vi "Write Status.vi"(5 "Username":string, 6 "Password":string, 7 "Address":string, 8 "Error In":errorcluster) -> (0 "Error Out":errorcluster)   [LabVIEW 2018, in "Tests.lvlib" / "SFTP File.lvlib"]
uses:
  SFTP File.lvlib
  src/Toolkit/SFTP File/Type Definitions/Open Options.ctl
  src/Toolkit/SFTP Attributes/Support/Create from SFTP File.vi
  src/Toolkit/SFTP Attributes/Support/Destroy to SFTP File.vi
  <vilib>/addons/_JKI Toolkits/Caraya/classes/Test/Test.lvclass
  <vilib>/addons/_JKI Toolkits/Caraya/classes/Assert/Assert.lvclass
  src/Toolkit/SFTP File/SFTP File.lvclass
  src/Toolkit/SFTP Attributes/SFTP Attributes.lvclass
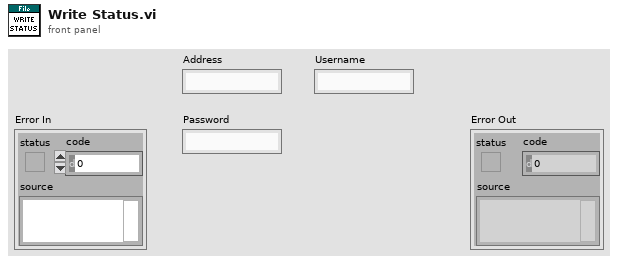
[diagram p1: front panel]
types:
  T1 = typedef "Toolkit.lvlib/SFTP File.lvclass/Open Options.ctl" = cluster{"Read":bool, "Write":bool, "Append":bool, "Create":bool, "Truncate":bool, "Exclude":bool}
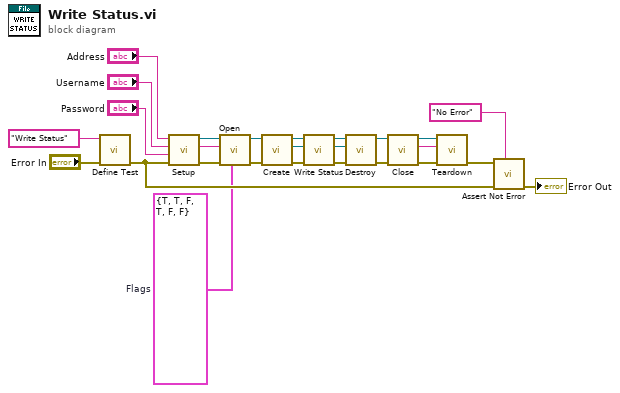
[diagram p0: block diagram]
diagram:
  w17 = T1 {"Read"=TRUE, "Write"=TRUE, "Append"=FALSE, "Create"=TRUE, "Truncate"=FALSE, "Exclude"=FALSE}  # Flags
  n1 = call <vilib>:"Define Test.vi"("error in (no error)"="Error In", "Label (VI Title)"="Write Status") -> ("error out"=w20:errorcluster)  [unwired: 9 in]
  n2 = call "Setup.vi"("Error In"=w20, "Password"="Password", "Username"="Username", "Address"="Address") -> ("Error Out"=w4:errorcluster, "Temporary File"=w5:string, "SFTP"=w18:refnum<class "SFTP.lvclass">)  [unwired: 5 in]
  n3 = call "Open.vi"("Flags"=w17, "Error In"=w4, "Remote Path"=w5, "SFTP"=w18) -> ("Error Out"=w15:errorcluster, "SFTP File"=w14:refnum<class "SFTP File.lvclass">)  [unwired: 6 in]
  n4 = call-poly "Create.vi"("Error In"=w15, "SFTP File In"=w14) -> ("Error Out"=w11:errorcluster, "SFTP Attributes"=w12:refnum<class "SFTP Attributes.lvclass">, "SFTP File Out"=w13:refnum<class "SFTP File.lvclass">)  [unwired: 7 in]
  n5 = call "Write Status.vi"("Error In"=w11, "Attributes In"=w12, "SFTP File In"=w13) -> ("Error Out"=w7:errorcluster, "Attributes Out"=w8:refnum<class "SFTP Attributes.lvclass">, "SFTP File Out"=w10:refnum<class "SFTP File.lvclass">)  [unwired: 6 in]
  n6 = call-poly "Destroy.vi"("Error In"=w7, "SFTP Attributes"=w8, "SFTP File In"=w10) -> ("Error Out"=w6:errorcluster, "SFTP File Out"=w9:refnum<class "SFTP File.lvclass">)  [unwired: 7 in]
  n7 = call "Close.vi"("Error In"=w6, "SFTP File"=w9) -> ("Error Out"=w1:errorcluster, "Remote Path"=w2:string, "SFTP"=w3:refnum<class "SFTP.lvclass">)  [unwired: 7 in]
  n8 = call "Teardown.vi"("Error In"=w1, "Temporary File"=w2, "SFTP"=w3) -> ("Error Out"=w19:errorcluster)  [unwired: 8 in]
  n9 = call <vilib>:"Assert Not Error.vi"("Label"="No Error", "error in (no error)"=w20, "Not Error?"=w19) -> ("error out"=→"Error Out":errorcluster)  [unwired: 8 in]
